vi "Process components.vi"(0 "Database Entry in":refnum<class "Database Entry.lvclass">, 5 "Do single-module data entry?":bool, 11 "error in (no error)":errorcluster) -> (1 "Status":string, 2 "Feet check":bool, 3 "PUT Settings":T1(array[cluster]), 4 "Database Entry out":refnum<class "Database Entry.lvclass">, 6 "Is real run?":bool, 7 "Module?":bool, 8 "Aborted":bool, 10 "Assembly Settings":T1(array[cluster]), 12 "Assembly Type":string[](array[string]), 13 "Stack names":string[](array[string]), 14 "Component Settings":T1(array[cluster]), 15 "error out":errorcluster)   [LabVIEW 2021, in "Database Entry.lvclass"]
uses:
  Database Entry.lvclass
  Database Entry.lvclass/Database Entry.ctl
  Components/Stack/Stack.lvclass
panel:
  out "Selected postitions":dbl[](array[numeric])
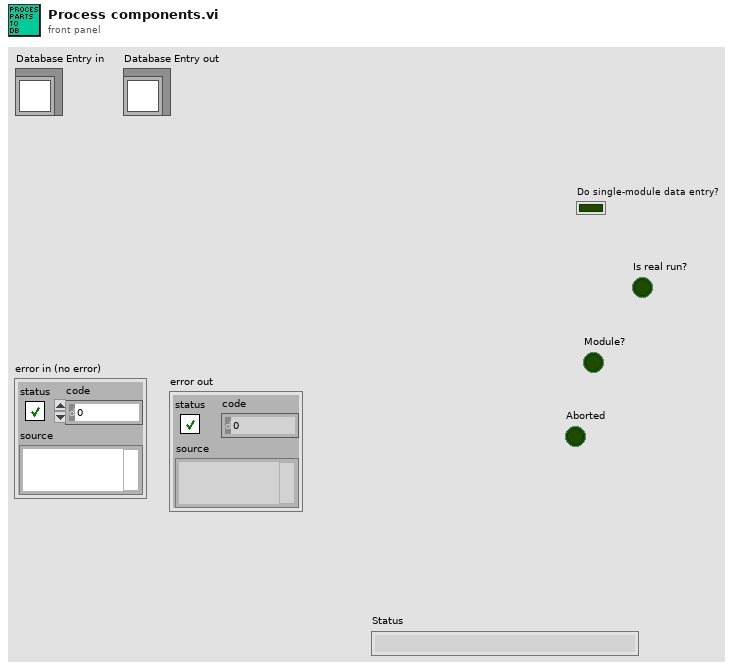
[diagram p1: front panel]
types:
  T1 = cluster{"Fixture ID":dbl, "Position":dbl, "Thickness":dbl}[]
  T2 = cluster{"Fixture ID":dbl, "Position":dbl, "Thickness":dbl}
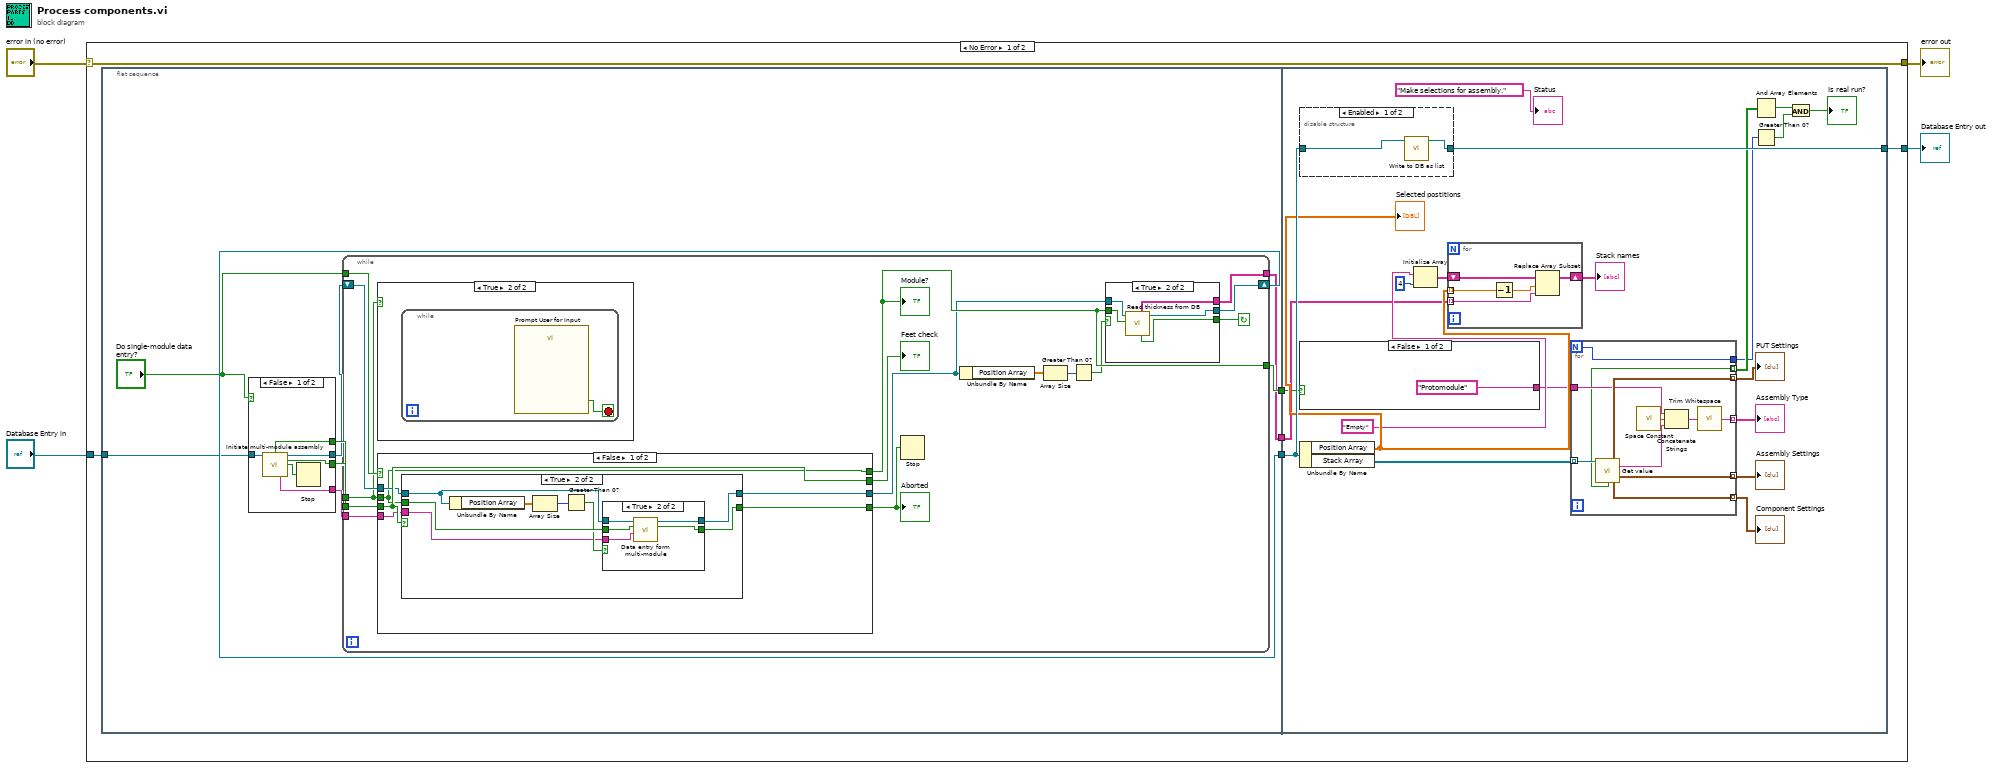
[diagram p0: block diagram]
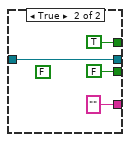
[diagram p2: hidden frame]
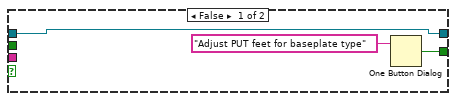
[diagram p4: hidden frame]
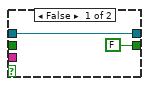
[diagram p5: hidden frame]
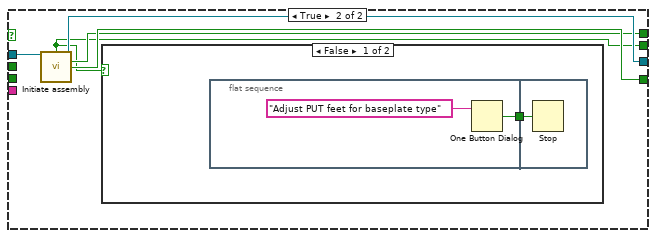
[diagram p6: hidden frame]
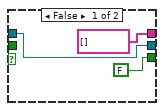
[diagram p8: hidden frame]
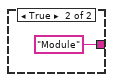
[diagram p9: hidden frame]
diagram:
  n1 = case shown="No Error" "error in (no error)" {
    selector: "error in (no error)" -> [w10 w130]
    tunnel: [w10 w130] -> w3
    tunnel: [w8 w129] -> w1
    tunnel: "Database Entry in" -> [w9 w129]
    frame No Error {
      n2 = flat-sequence {
        tunnel: [w19] -> w7
        tunnel: [w17] -> w6
        tunnel: [w18] -> w5
        tunnel: w9 -> [w15]
        tunnel: w7 -> [w102]
        tunnel: [w100] -> w8
        tunnel: w6 -> [w94]
        tunnel: w5 -> [w93]
        frame #0 {
          n3 = case shown="False" "Do single-module data entry?" {
            tunnel: w15 -> [w23 w29]
            tunnel: [w22 w29] -> w12
            tunnel: [w25 TRUE ("Feet check")] -> w14
            tunnel: [w24 FALSE ("Module?")] -> w13
            tunnel: [w20 "" ("Module type out")] -> w11
            frame False {
              n4 = call "Initiate multi-module assembly.vi"("Database Entry in"=w23) -> ("Feet check"=w25:bool, "Database Entry out"=w22:refnum<class "Database Entry.lvclass">, "Module?"=w24:bool, "Abort out"=w21:bool, "Module type out"=w20:string)  [unwired: 9 in, 1 out]
              n5 = Stop(stop? (T)=w21) -> ()
            }
            frame True {
              (unwired) FALSE ("Abort out")
            }
          }
          n6 = while {
            tunnel: [w38] -> w17
            shift-right: [w44] -> w19
            shift-left: w12 -> [w37]
            tunnel: "Do single-module data entry?" -> [w34]
            tunnel: [w43] -> w18
            tunnel: w14 -> [w32]
            tunnel: w13 -> [w30]
            tunnel: w11 -> [w31]
            stop <- w33 continue-if-true
            n7 = case shown="True" w30 {
              frame False {
              }
              frame True {
                n8 = while {
                  stop <- w45 stop-if-true
                  n9 = call "Prompt User for Input"() -> ("Hexaboards ready?"=w45:bool)  [unwired: 17 in, 2 out]
                }
              }
            }
            n10 = case shown="False" w34 {
              tunnel: w37 -> [w48 w74]
              tunnel: [w51 w73] -> w42
              tunnel: [w49 w70] -> w36
              tunnel: [w50 w72] -> w35
              tunnel: [w47 w71] -> w43
              tunnel: w32 -> [w49 _]
              tunnel: w30 -> [w47 _]
              tunnel: w31 -> [w46 _]
              frame False {
                n11 = case shown="True" w49 {
                  tunnel: w47 -> [_ w62]
                  tunnel: w48 -> [w54 w59]
                  tunnel: [w54 w61] -> w51
                  tunnel: [w52 w60] -> w50
                  tunnel: w46 -> [_ w55]
                  frame False {
                    n12 = One Button Dialog(message="Adjust PUT feet for baseplate type") -> (true=w52:bool)  [unwired: 1 in]
                  }
                  frame True {
                    n13 = Unbundle By Name(w59) -> ("Position Array"=w58:dbl[])
                    n14 = Array Size(array=w58) -> (size(s)=w57:i32)
                    n15 = Greater Than 0?(x=w57) -> (x > 0?=w56:bool)
                    n16 = case shown="True" w56 {
                      tunnel: w62 -> [_ w69]
                      tunnel: [w64 w68] -> w61
                      tunnel: [FALSE ("Aborted") w67] -> w60
                      tunnel: w59 -> [w64 w66]
                      tunnel: w55 -> [_ w65]
                      frame False {
                      }
                      frame True {
                        n17 = call "Data entry form multi-module.vi"("Assembly Type"=w65, "Is Module?"=w69, "Database Entry in"=w66) -> ("Aborted"=w67:bool, "Database Entry out"=w68:refnum<class "Database Entry.lvclass">)  [unwired: 5 in, 2 out]
                      }
                    }
                  }
                }
              }
              frame True {
                n18 = call "Initiate assembly.vi"("Database Entry in"=w74) -> ("Feet check"=w70:bool, "Database Entry out"=w73:refnum<class "Database Entry.lvclass">, "Module?"=w71:bool, "Abort out"=w72:bool)  [unwired: 10 in, 1 out]
                n19 = case shown="False" w70 {
                  frame False {
                    n20 = flat-sequence {
                      tunnel: [w76] -> w75
                      tunnel: w75 -> [w78]
                      frame #0 {
                        n21 = One Button Dialog(message="Adjust PUT feet for baseplate type") -> (true=w76:bool)  [unwired: 1 in]
                      }
                      frame #1 {
                        n22 = Stop(stop? (T)=w78) -> ()
                      }
                    }
                  }
                  frame True {
                  }
                }
              }
            }
            "Module?" <- w43
            "Aborted" <- w35
            "Feet check" <- w36
            n23 = Stop(stop? (T)=w35) -> ()
            n24 = Unbundle By Name(w42) -> ("Position Array"=w41:dbl[])
            n25 = Array Size(array=w41) -> (size(s)=w40:i32)
            n26 = Greater Than 0?(x=w40) -> (x > 0?=w39:bool)
            n27 = case shown="True" w39 {
              tunnel: [w81 w86] -> w44
              tunnel: w43 -> [_ w85]
              tunnel: w42 -> [w81 w84]
              tunnel: [string[] [] w83] -> w38
              tunnel: [FALSE ("Change parts") w82] -> w33
              frame False {
              }
              frame True {
                n28 = call "Read thickness from DB.vi"("Module?"=w85, "Database Entry in"=w84) -> ("Database Entry out"=w86:refnum<class "Database Entry.lvclass">, "Replace parts"=w82:bool, "Stack names"=w83:string[])  [unwired: 4 in, 3 out]
              }
            }
          }
        }
        frame #1 {
          n29 = disable-structure shown="Enabled" {
            disable-tunnel: w102 -> [w111 w112]
            disable-tunnel: [w110 w112] -> w100
            frame Enabled {
              n30 = call "Write to DB as list.vi"("Database Entry in"=w111) -> ("Database Entry out"=w110:refnum<class "Database Entry.lvclass">)  [unwired: 8 in, 2 out]
            }
            frame Disabled {
            }
          }
          n31 = case shown="False" w93 {
            tunnel: ["Protomodule" "Module"] -> w92
            frame False {
            }
            frame True {
            }
          }
          n32 = Unbundle By Name(w102) -> ("Position Array"=w101:dbl[], "Stack Array"=w107:refnum<class "Stack.lvclass">[])
          "Selected postitions" <- w101
          n33 = Initialize Array("Empty", 4 ("dimension size")) -> (w96:string[])
          n34 = for {
            tunnel: w101 -> [w115] mode=indexing
            tunnel: w94 -> [w116] mode=indexing
            shift-right: [w113] -> w99
            shift-left: w96 -> [w117]
            n35 = Decrement(x=w115) -> (x-1=w114:dbl)
            n36 = Replace Array Subset(array=w117, new element=w116, index=w114) -> (w113:string[])
          }
          "Stack names" <- w99
          n37 = for {
            N -> [w120]
            tunnel: w107 -> [w128] mode=indexing
            tunnel: [w127] -> w106 mode=indexing
            tunnel: [w125] -> w105 mode=indexing
            tunnel: [w126] -> w104 mode=indexing
            tunnel: [w118] -> w103 mode=indexing
            tunnel: w92 -> [w122]
            tunnel: [w121] -> w91 mode=indexing
            tunnel: [w120] -> w90
            n38 = call "Get value.vi"("Stack in"=w128) -> ("PUT Settings"=w127:T2, "Resolution Geometry"=w124:string, "Assembly Settings"=w126:T2, "Is real run"=w121:bool, "Component Settings"=w125:T2)  [unwired: 8 in, 2 out]
            n39 = call <vilib>:"Space Constant.vi"() -> ("String"=w123:string)
            n40 = Concatenate Strings(w122, w123, w124) -> (w119:string)
            n41 = call <vilib>:"Trim Whitespace.vi"("string"=w119) -> ("trimmed string"=w118:string)  [unwired: 1 in]
          }
          "Assembly Settings" <- w104
          "Component Settings" <- w105
          "PUT Settings" <- w106
          "Assembly Type" <- w103
          n42 = And Array Elements(Boolean array=w91) -> (logical AND=w88:bool)
          n43 = Greater Than 0?(x=w90) -> (x > 0?=w89:bool)
          n44 = And(x=w88, y=w89) -> (x .and. y?=→"Is real run?":bool)
          "Status" <- "Make selections for assembly." ("Status")
        }
      }
    }
    frame Error {
    }
  }
  "error out" <- w3
  "Database Entry out" <- w1
